vi "Send Command.vi"(8 "error in (no error)":errorcluster, 10 "write buffer":string, 11 "VISA resource name":refnum<visa-resource-name>) -> (0 "error out":errorcluster, 3 "VISA resource name out":refnum<visa-resource-name>)   [LabVIEW 2017, in "JY-SPEX-TRIAX.lvlib"]
doc: "Sends the given command to the spectrometer (and uses semaphores to make sure of exclusive access)."
uses:
  JY-SPEX-TRIAX.lvlib
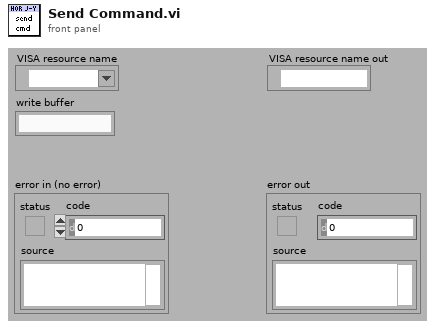
[diagram p1: front panel]
types:
  T1 = typedef "Semaphore RefNum" = refnum<k1>
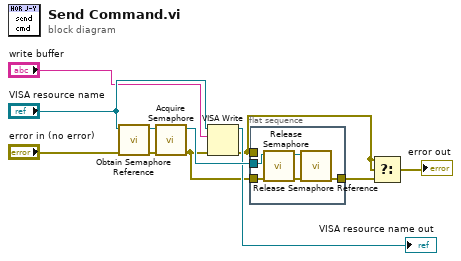
[diagram p0: block diagram]
diagram:
  n1 = call <vilib>:"Obtain Semaphore Reference.vi"("error in (no error)"="error in (no error)", "name (unnamed)"="VISA resource name") -> ("error out"=w11:errorcluster, "semaphore"=w8:T1)  [unwired: 1 in, 3 out]
  n2 = call <vilib>:"Acquire Semaphore.vi"("error in (no error)"=w11, "semaphore"=w8) -> ("error out"=w2:errorcluster, "semaphore out"=w7:T1)  [unwired: 1 in, 3 out]
  n3 = VISA Write(VISA resource name="VISA resource name", write buffer="write buffer", error in (no error)=w2) -> (VISA resource name out=→"VISA resource name out":refnum<visa-resource-name>, error out=w1:errorcluster)  [unwired: 1 out]
  n4 = flat-sequence {
    tunnel: w7 -> [w16]
    tunnel: [w13] -> w4
    tunnel: w2 -> [w12]
    tunnel: w1 -> [_]
    frame #0 {
      n5 = call <vilib>:"Release Semaphore.vi"("error in (no error)"=w12, "semaphore"=w16) -> ("error out"=w15:errorcluster, "semaphore out"=w14:T1)  [unwired: 4 out]
      n6 = call <vilib>:"Release Semaphore Reference.vi"("error in (no error)"=w15, "semaphore"=w14) -> ("error out"=w13:errorcluster)  [unwired: 9 out]
    }
  }
  n7 = Select(t=w1, s=w1, f=w4) -> (s? t:f=→"error out":errorcluster)
